vi "4D Grapher.vi"(4 "Norm Factor (NaN: use first element)":dbl format="%#_13g", 6 "Normalize? (F)":bool, 8 "Pruned Data":string[][](array[string]), 9 "String Items from Axes Menus":cluster{string[]}[](array[cluster]), 10 "Axes Indexes":i32[](array[numeric]), 11 "Axes Names":string[](array[string])) -> (0 "Graph":T2(array[cluster]), 3 "Color Axis Titles":string[](array[string]))   [LabVIEW 2019]
uses:
  AxisMenu--Enum.ctl
  <vilib>/Analysis/baseanly.llb/Mean (DBL).vi
  <vilib>/Analysis/NI_AALBase.lvlib
panel:
  in  "Axis Menu Type Def":T1 caption="Axis Menu" items=["<Ignore>", "<X Axis>", "<Y Axis>", "<Color Axis>", "<Time Axis>", "<Supra-X Scroll>", "<Supra-Y Scroll>"]
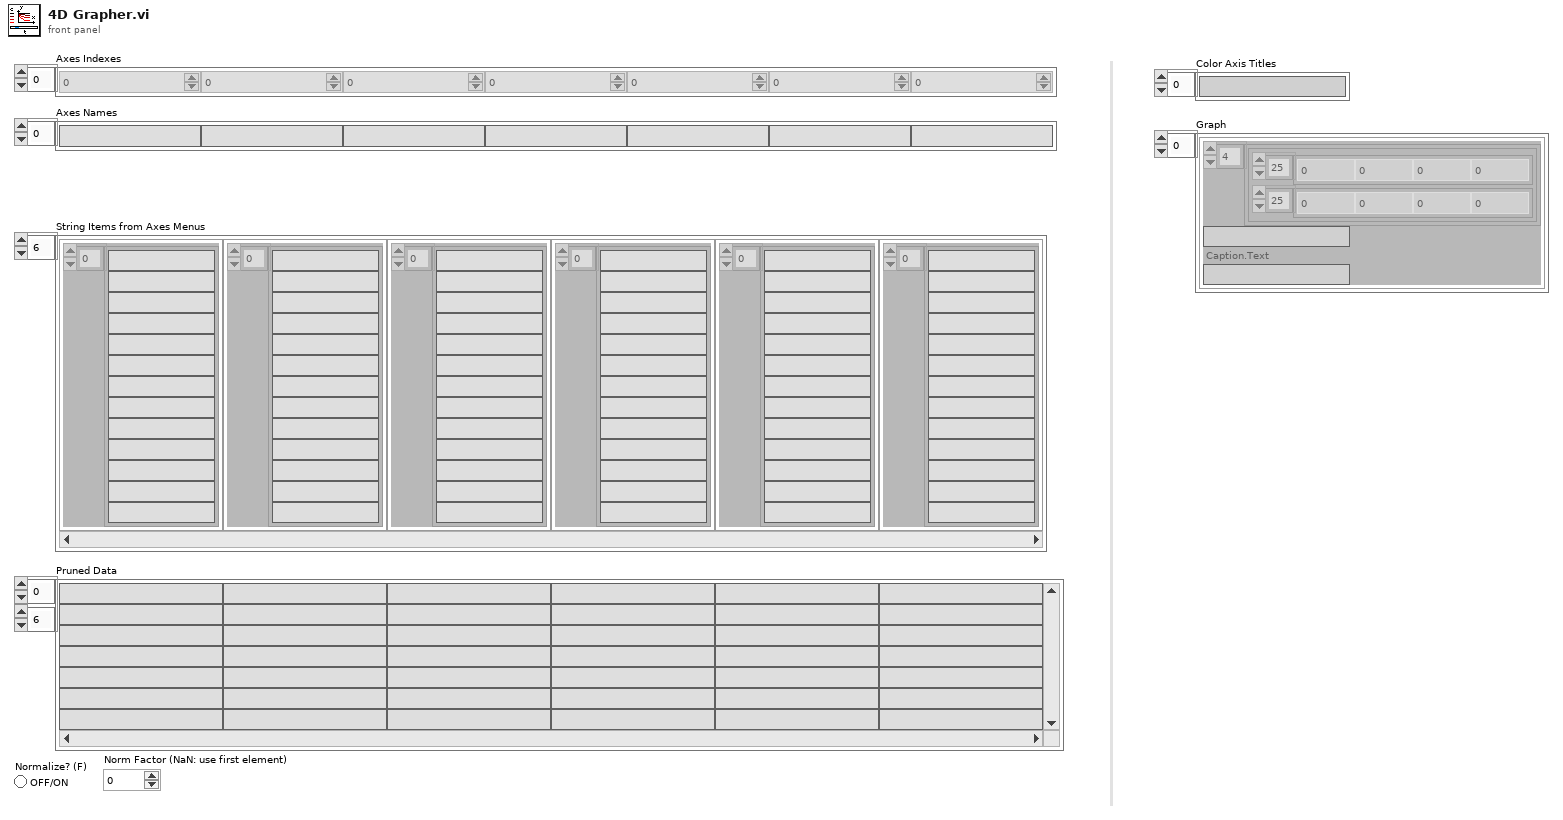
[diagram p1: front panel]
types:
  T1 = typedef "AxisMenu--Enum.ctl" = u16
  T2 = cluster{cluster{dbl[], dbl[]}[], string, "Caption.Text":string}[]
  T3 = cluster{cluster{dbl[], dbl[]}[], string, string}[]
  T4 = cluster{dbl, cluster{dbl[], dbl[]}[], string, "Caption.Text":string}
  T5 = cluster{dbl, cluster{dbl[], dbl[]}[], string, "Caption.Text":string}[]
  T6 = cluster{cluster{dbl[], dbl[]}[], string, "Caption.Text":string}
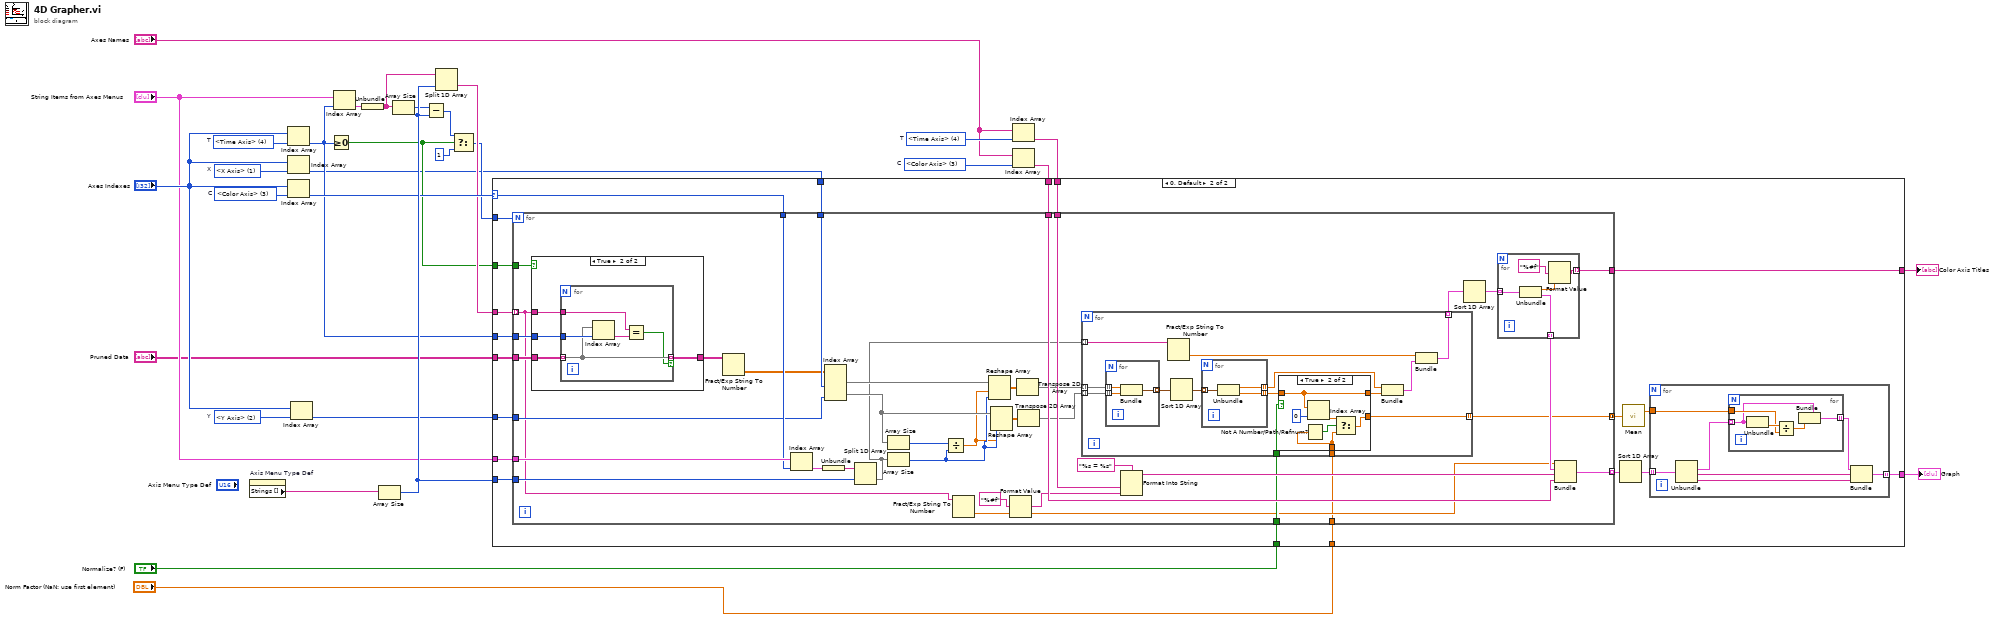
[diagram p0: block diagram]
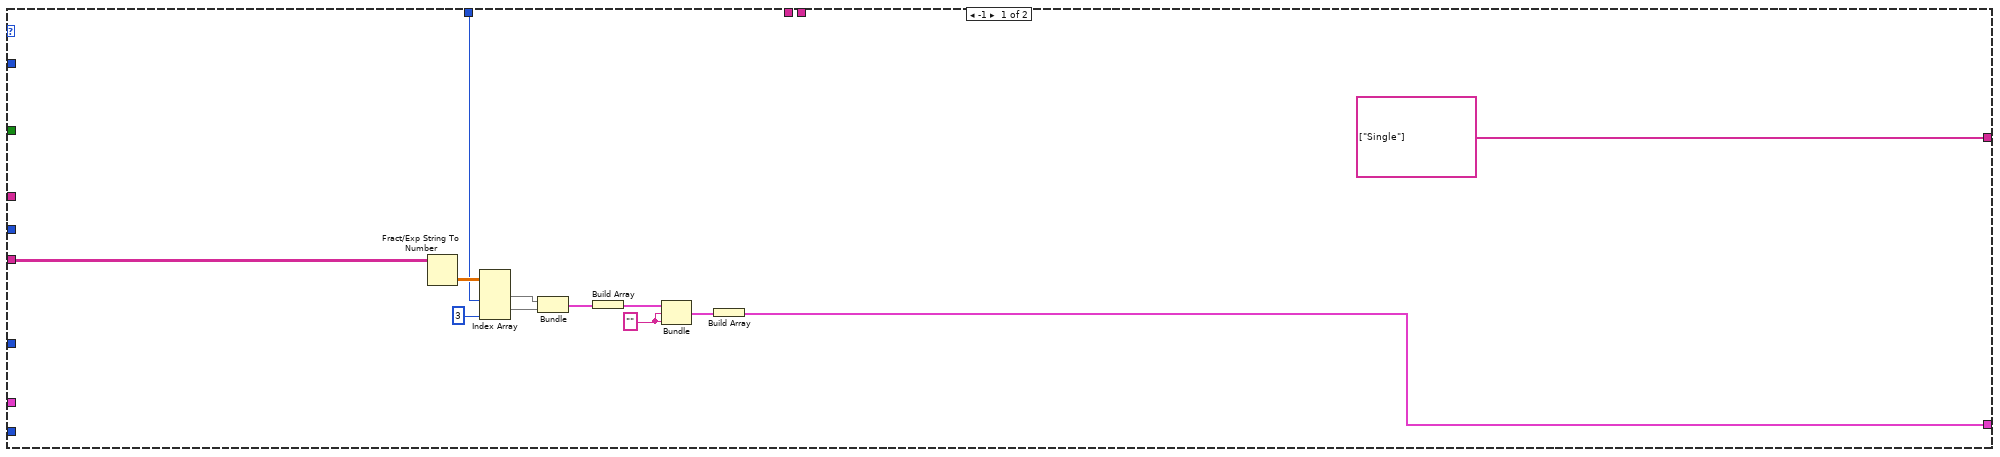
[diagram p2: hidden frame]
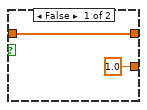
[diagram p4: hidden frame]
diagram:
  w29 = T1 3 items=["<Ignore>", "<X Axis>", "<Y Axis>", "<Color Axis>", "<Time Axis>", "<Supra-X Scroll>", "<Supra-Y Scroll>"]  # C
  w28 = T1 4 items=["<Ignore>", "<X Axis>", "<Y Axis>", "<Color Axis>", "<Time Axis>", "<Supra-X Scroll>", "<Supra-Y Scroll>"]  # T
  w22 = T1 3 items=["<Ignore>", "<X Axis>", "<Y Axis>", "<Color Axis>", "<Time Axis>", "<Supra-X Scroll>", "<Supra-Y Scroll>"]  # C
  w21 = T1 1 items=["<Ignore>", "<X Axis>", "<Y Axis>", "<Color Axis>", "<Time Axis>", "<Supra-X Scroll>", "<Supra-Y Scroll>"]  # X
  w20 = T1 4 items=["<Ignore>", "<X Axis>", "<Y Axis>", "<Color Axis>", "<Time Axis>", "<Supra-X Scroll>", "<Supra-Y Scroll>"]  # T
  w19 = T1 2 items=["<Ignore>", "<X Axis>", "<Y Axis>", "<Color Axis>", "<Time Axis>", "<Supra-X Scroll>", "<Supra-Y Scroll>"]  # Y
  n1 = property on="Axis Menu Type Def" class="Ring (strict)"() -> ("Strings []"=w2:string[])  [unwired: 2 in, 2 out]
  n2 = Index Array(array="Axes Indexes", index=w20) -> (element=w13:i32)
  n3 = Index Array(array="Axes Indexes", index=w21) -> (element=w4:i32)
  n4 = Index Array(array="Axes Indexes", index=w22) -> (element=w15:i32)
  n5 = Index Array(array="Axes Indexes", index=w19) -> (element=w17:i32)
  n6 = Greater Or Equal To 0?(x=w13) -> (x >= 0?=w10:bool)
  n7 = Index Array(array="String Items from Axes Menus", index=w13) -> (element=w5:cluster{string[]})
  n8 = Unbundle(w5) -> (w11:string[])
  n9 = Array Size(array=w2) -> (size(s)=w30:i32)
  n10 = Array Size(array=w11) -> (size(s)=w6:i32)
  n11 = Subtract(x=w6, y=w30) -> (x-y=w7:i32)
  n12 = Split 1D Array(array=w11, index=w30) -> (second subarray=w12:string[])  [unwired: 1 out]
  n13 = Select(t=w7, s=w10, f=1) -> (s? t:f=w9:i32)
  n14 = Index Array(array="Axes Names", index=w28) -> (element=w26:string)
  n15 = Index Array(array="Axes Names", index=w29) -> (element=w25:string)
  n16 = case shown="0, Default" w15 {
    selector: w15 -> [_ w59]
    tunnel: "Pruned Data" -> [w38 w62]
    tunnel: w4 -> [w37 w61]
    tunnel: "String Items from Axes Menus" -> [_ w60]
    tunnel: [string[] ["Single"] w58] -> w3
    tunnel: w30 -> [_ w57]
    tunnel: w9 -> [_ w56]
    tunnel: [w31 w46] -> w14
    tunnel: w12 -> [_ w54]
    tunnel: w10 -> [_ w53]
    tunnel: w13 -> [_ w52]
    tunnel: w26 -> [_ w51]
    tunnel: w25 -> [_ w50]
    tunnel: w17 -> [_ w48]
    tunnel: "Normalize? (F)" -> [_ w49]
    tunnel: "Norm Factor (NaN: use first element)" -> [_ w43]
    frame -1 {
      w33 = ""
      n17 = Fract/Exp String To Number(string=w38) -> (number=w40:dbl[][])  [unwired: 3 in, 1 out]
      n18 = Index Array(array=w40, index (col) #1=w37, index (col) #2=3 ("index (col)")) -> (element #1=w41:dbl[], element #2=w42:dbl[])  [unwired: 2 in]
      n19 = Bundle(w41, w42) -> (w36:cluster{dbl[], dbl[]})  [unwired: 1 in]
      n20 = Build Array(w36) -> (w34:cluster{dbl[], dbl[]}[])
      n21 = Bundle(w34, w33, w33) -> (w32:cluster{cluster{dbl[], dbl[]}[], string, string})  [unwired: 1 in]
      n22 = Build Array(w32) -> (w31:T3)
    }
    frame 0, Default {
      n23 = for {
        N: w56 -> [_]
        tunnel: w62 -> [w91]
        tunnel: w61 -> [w100]
        tunnel: w60 -> [w98]
        tunnel: w59 -> [w97]
        tunnel: [w70] -> w58
        tunnel: w57 -> [w94]
        tunnel: [w93] -> w55 mode=indexing
        tunnel: w54 -> [w68] mode=indexing
        tunnel: w53 -> [w92]
        tunnel: w52 -> [w89]
        tunnel: w51 -> [w88]
        tunnel: w50 -> [w85]
        tunnel: w48 -> [w84]
        tunnel: w49 -> [w69]
        tunnel: [w64] -> w45 mode=concatenating
        tunnel: w43 -> [w63]
        n24 = case shown="True" w92 {
          tunnel: w91 -> [w106 w110]
          tunnel: [w106 w107] -> w90
          tunnel: w68 -> [_ w108]
          tunnel: w89 -> [_ w109]
          frame False {
          }
          frame True {
            n25 = for {
              tunnel: w110 -> [w112] mode=indexing
              tunnel: w109 -> [w115]
              tunnel: w108 -> [w114]
              tunnel: [w112] -> w107 mode=indexing if=w111
              n26 = Index Array(array=w112, index=w115) -> (element=w113:string)
              n27 = Equal?(x=w114, y=w113) -> (x = y?=w111:bool)
            }
          }
        }
        n28 = Fract/Exp String To Number(string=w90) -> (number=w81:dbl[][])  [unwired: 3 in, 1 out]
        n29 = Index Array(array=w98, index=w97) -> (element=w96:cluster{string[]})
        n30 = Unbundle(w96) -> (w95:string[])
        n31 = Index Array(array=w81, index (col) #1=w100, index (col) #2=w84) -> (element #1=w83:dbl[], element #2=w82:dbl[])  [unwired: 2 in]
        n32 = Split 1D Array(array=w95, index=w94) -> (second subarray=w71:string[])  [unwired: 1 out]
        n33 = Array Size(array=w82) -> (size(s)=w99:i32)
        n34 = Array Size(array=w71) -> (size(s)=w78:i32)
        n35 = Divide(x=w99, y=w78) -> (x/y=w77:dbl)
        n36 = Fract/Exp String To Number(string=w68) -> (number=w65:dbl)  [unwired: 3 in, 1 out]
        n37 = Reshape Array(w83, w77, w78) -> (w80:dbl[][])
        n38 = Reshape Array(w82, w77, w78) -> (w79:dbl[][])
        n39 = Format Value(format string="%#f", value (0)=w65) -> (output string=w66:string)  [unwired: 1 in]
        n40 = Transpose 2D Array(2D array=w80) -> (transposed array=w76:dbl[][])
        n41 = Transpose 2D Array(2D array=w79) -> (transposed array=w75:dbl[][])
        n42 = for {
          tunnel: w75 -> [w125] mode=indexing
          tunnel: w76 -> [w126] mode=indexing
          tunnel: w71 -> [w122] mode=indexing
          tunnel: [w119] -> w74 mode=indexing
          tunnel: w69 -> [w118]
          tunnel: [w117] -> w64 mode=indexing
          tunnel: w63 -> [w116]
          n43 = for {
            tunnel: w126 -> [w143] mode=indexing
            tunnel: w125 -> [w142] mode=indexing
            tunnel: [w141] -> w129 mode=indexing
            n44 = Bundle("String"=w143, "String"=w142) -> (w141:cluster{"String":dbl, "String":dbl})  [unwired: 1 in]
          }
          n45 = Fract/Exp String To Number(string=w122) -> (number=w121:dbl)  [unwired: 3 in, 1 out]
          n46 = Sort 1D Array(array=w129) -> (sorted array=w128:cluster{"String":dbl, "String":dbl}[])
          n47 = for {
            tunnel: w128 -> [w140] mode=indexing
            tunnel: [w139] -> w127 mode=indexing
            tunnel: [w138] -> w124 mode=indexing
            n48 = Unbundle(w140) -> ("String"=w139:dbl, "String"=w138:dbl)
          }
          n49 = case shown="True" w118 {
            tunnel: w124 -> [w131 w136]
            tunnel: [w131 w136] -> w123
            tunnel: [1.0 ("String") w134] -> w117
            tunnel: w116 -> [_ w133]
            frame False {
            }
            frame True {
              n50 = Not A Number/Path/Refnum?(number/path/refnum=w133) -> (NaN/Path/Refnum?=w132:bool)
              n51 = Index Array(array=w136, index=0) -> (element=w135:dbl)
              n52 = Select(t=w135, s=w132, f=w133) -> (s? t:f=w134:dbl)
            }
          }
          n53 = Bundle(w127, w123) -> (w120:cluster{dbl[], dbl[]})  [unwired: 1 in]
          n54 = Bundle(w121, w120) -> (w119:cluster{dbl, cluster{dbl[], dbl[]}})  [unwired: 1 in]
        }
        n55 = Format Into String(format string="%s = %s", w88, w66) -> (resulting string=w87:string)  [unwired: 2 in, 1 out]
        n56 = Sort 1D Array(array=w74) -> (sorted array=w73:cluster{dbl, cluster{dbl[], dbl[]}}[])
        n57 = for {
          tunnel: w73 -> [w105] mode=indexing
          tunnel: [w104] -> w72 mode=indexing
          tunnel: [w101] -> w70 mode=indexing
          n58 = Unbundle(w105) -> (w102:dbl, w104:cluster{dbl[], dbl[]})
          n59 = Format Value(format string="%#f", value (0)=w102) -> (output string=w101:string)  [unwired: 1 in]
        }
        n60 = Bundle(w65, w72, w87, "Caption.Text"=w85) -> (w93:T4)  [unwired: 1 in]
      }
      n61 = Sort 1D Array(array=w55) -> (sorted array=w47:T5)
      n62 = call-poly <vilib>:"Mean.vi"("X"=w45) -> ("mean"=w44:dbl)  [unwired: 1 out]
      n63 = for {
        tunnel: w47 -> [w150] mode=indexing
        tunnel: [w147] -> w46 mode=indexing
        tunnel: w44 -> [w146]
        n64 = Unbundle(w150) -> (w145:cluster{dbl[], dbl[]}[], w149:string, "Caption.Text"=w148:string)  [unwired: 1 out]
        n65 = for {
          tunnel: w145 -> [w153] mode=indexing
          tunnel: w146 -> [w154]
          tunnel: [w151] -> w144 mode=indexing
          n66 = Unbundle(w153) -> (w155:dbl[])  [unwired: 1 out]
          n67 = Divide(x=w155, y=w154) -> (x/y=w152:dbl[])
          n68 = Bundle(cluster=w153, w152) -> (w151:cluster{dbl[], dbl[]})  [unwired: 1 in]
        }
        n69 = Bundle(w144, w149, "Caption.Text"=w148) -> (w147:T6)  [unwired: 1 in]
      }
    }
  }
  "Graph" <- w14
  "Color Axis Titles" <- w3
